vi "High Bee.vi"   [LabVIEW 2020]
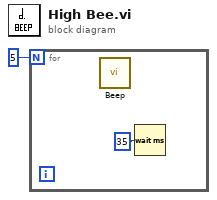
[diagram p0: block diagram]
diagram:
  n1 = for {
    N: 5 -> [_]
    n2 = call <vilib>:"Beep.vi"() -> ()  [unwired: 12 in]
    n3 = Wait (ms)(milliseconds to wait=35) -> ()  [unwired: 1 out]
  }
